vi "Read Model Number.vi"(0 "Error In":errorcluster) -> (1 "Target Info":T1, 2 "Error Out":errorcluster)   [LabVIEW 2018]
uses:
  <vilib>/nisyscfg/Close (System).vi
  <vilib>/nisyscfg/nisyscfg.lvlib
  <resource>/objmgr/nisysapi.rc
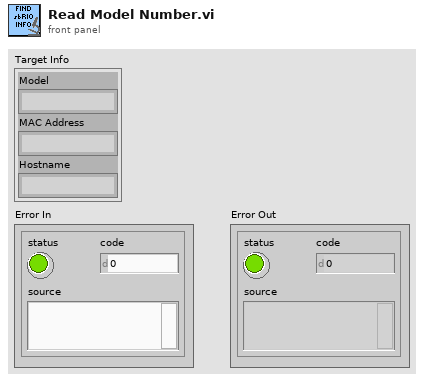
[diagram p1: front panel]
types:
  T1 = cluster{"Model":string, "MAC Address":string, "Hostname":string}
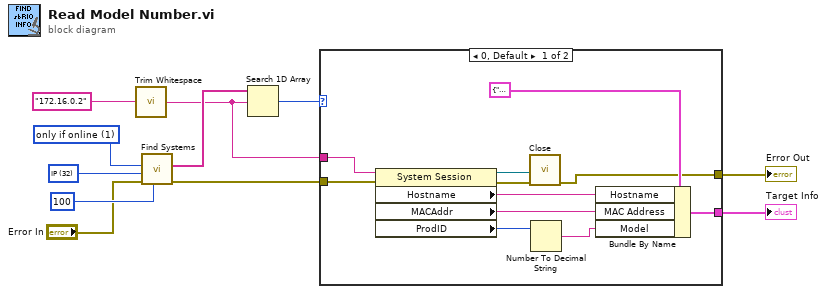
[diagram p0: block diagram]
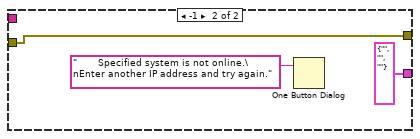
[diagram p2: hidden frame]
diagram:
  w10 = u32 32 items=["Hostname"=16, "Hostname (IP)"=18, "Hostname (MAC)"=19, "IP"=32, "IP (Hostname)"=33, "IP (MAC)"=35, "MAC"=48, "MAC (Hostname)"=49, "MAC (IP)"=50] ("Output (Hostname and IP)")
  w11 = u32 1 items=["none"=0, "only if online"=1, "all"=3] ("Include Cached Results (all)")
  n1 = call <vilib>:"Trim Whitespace.vi"("string"="172.16.0.2" ("IP Address")) -> ("trimmed string"=w1:string)  [unwired: 1 in]
  n2 = call <vilib>:"Find Systems.vi"("Timeout (4000 ms)"=u32 100, "error in (no error)"="Error In", "Output (Hostname and IP)"=w10, "Include Cached Results (all)"=w11) -> ("error out"=w6:errorcluster, "Detected Systems"=w5:string[])  [unwired: 5 in, 1 out]
  n3 = Search 1D Array(1D array=w5, element=w1) -> (index of element=w7:i32)  [unwired: 1 in]
  n4 = case shown="0, Default" w7 {
    tunnel: w6 -> [w22 w24]
    tunnel: w1 -> [w20 _]
    tunnel: [w15 T1 {"Model"="", "MAC Address"="", "Hostname"=""} ("input cluster")] -> w4
    tunnel: [w12 w24] -> w3
    frame 0, Default {
      n5 = property class="System Session"(reference=w20, error in=w22) -> (reference out=w19:refnum<k21>, error out=w21:errorcluster, "Hostname"=w17:string, "MACAddr"=w16:string, "ProdID"=w14:i32)
      n6 = call-poly <vilib>:"Close.vi"("error in (no error)"=w21, "Session in"=w19) -> ("error out"=w12:errorcluster)  [unwired: 9 in]
      n7 = Number To Decimal String(number=w14) -> (decimal integer string=w13:string)  [unwired: 1 in]
      n8 = Bundle By Name(cluster=T1 {"Model"="", "MAC Address"="", "Hostname"=""} ("input cluster"), "Hostname"=w17, "MAC Address"=w16, "Model"=w13) -> (w15:T1)
    }
    frame -1 {
      n9 = One Button Dialog(message="       Specified system is not online.\nEnter another IP address and try again.") -> ()  [unwired: 1 in, 1 out]
    }
  }
  "Error Out" <- w3
  "Target Info" <- w4
